vi "Spline Interpolation.vi"(2 "x value":dbl format="%0.2f", 3 "Interpolant":dbl[](array[numeric]) format="%0.2f", 4 "X":dbl[](array[numeric]) format="%0.2f", 5 "Y":dbl[](array[numeric]) format="%0.2f") -> (0 "error":i32, 1 "interpolation value":dbl format="%0.2f")   [LabVIEW 2017, in "NI_AALPro.lvlib"]
doc: "Returns a spline interpolated value at <B>x value</B> given the tabulated values (x[i], y[i]) and the second derivatives <B>Interpolant</B> that the VI obtains from the Spline Interpolant VI."
uses:
  <vilib>/Analysis/NI_AALPro.lvlib
  <resource>/lvanlys.dll
panel:
  # "Spline Interpolation"
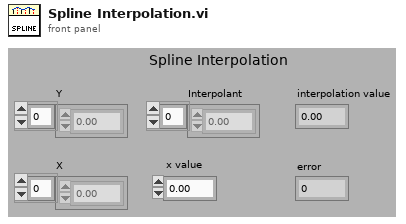
[diagram p1: front panel]
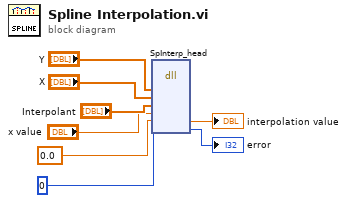
[diagram p0: block diagram]
diagram:
  n1 = dll-call lib="e:/builds/penguin/labview/branches/2017/dev/dist/resource/lvanlys.*" fn="SpInterp_head"("Y"="Y", "X"="X", "Interpolant"="Interpolant", "x value"="x value", "output param"=0.0, "output param"=0) -> ("output param"=→"interpolation value":dbl, "output param"=→"error":i32)  [unwired: 8 in, 2 out]
